vi "Teleop.vi"(10 "Match Info":T1={"Autonomous Elapsed Seconds"=0.0, "TeleOp Elapsed Seconds"=0.0, "Disabled Elapsed Seconds"=0.0, "Visited Autonomous"=FALSE, "Visited TeleOp"=FALSE, "Visited Disabled"=FALSE, "Autonomous Settings"={"Autonomous Style"=enum."Independent", "VI Refnum"=refnum}}, 11 "Call Context":T2) -> ()   [LabVIEW 2017]
doc: "This VI is called for each enabled TeleOp packet received from the DS. It is typically used to read from joysticks and other inputs and update I/O or setpoints for timed control loops. It should complete and return within 20 milliseconds or risk missing DS packets."
uses:
  <vilib>/Rock Robotics/WPI/DriverStation/WPI_DriverStationDerivedRobotMode.ctl
  <vilib>/Rock Robotics/WPI/DriverStation/WPI_DriverStationMatch Info.ctl
  <vilib>/Rock Robotics/WPI/Relay/WPI_RelayValue.ctl
  <vilib>/Rock Robotics/WPI/Solenoid/WPI_SolenoidValue.ctl
  <vilib>/Rock Robotics/WPI/Utilities/WPI_GetSetVariantRefNum.vi
  <vilib>/Rock Robotics/WPI/RobotDrive/WPI_RobotDriveMecanumDrive_Cartesian.vi
  <vilib>/Rock Robotics/WPI/Solenoid/WPI_SolenoidSetEnum.vi
panel:
  out "Distance":dbl
  out "Magnet sensed 2":bool
  out "Magnet sensed 1":bool
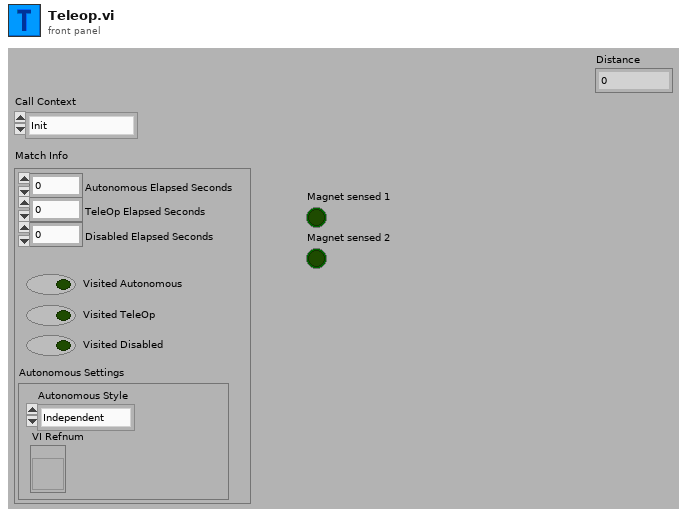
[diagram p1: front panel]
types:
  T1 = typedef "WPI_DriverStationMatch Info.ctl" = cluster{"Autonomous Elapsed Seconds":dbl, "TeleOp Elapsed Seconds":dbl, "Disabled Elapsed Seconds":dbl, "Visited Autonomous":bool, "Visited TeleOp":bool, "Visited Disabled":bool, "Autonomous Settings":cluster{"Autonomous Style":enum16{"Iterative", "Independent"}, "VI Refnum":refnum<vi>}}
  T2 = typedef "WPI_DriverStationDerivedRobotMode.ctl" = enum16{"Init", "Execute", "Stop"}
  T3 = typedef "WPI_SolenoidValue.ctl" = enum16{"Off", "On", "Forward", "Reverse"}
  T4 = typedef "WPI_RelayValue.ctl" = enum16{"Off", "On", "Forward", "Reverse"}
  T5 = typedef "WPI_CompressorDevRef.ctl" = cluster{"DevStatus":errorcluster, "Pneumatics Control Module":u8}
  T6 = typedef "WPI_EncoderDevRef.ctl" = cluster{"DevStatus":errorcluster, "EncoderIndex":T7, "CounterIndex":T8, "DistancePerCount":dbl, "Decoding Type":T9}
  T7 = typedef "FPGA_EncoderIdx.ctl" = enum8{"Enc 0", "Enc 1", "Enc 2", "Enc 3", "Enc 4", "Enc 5", "Enc 6", "Enc 7", "Invalid"}
  T8 = typedef "FPGA_CounterCtrSystemIndex.ctl" = enum8{"Ctr 0", "Ctr 1", "Ctr 2", "Ctr 3", "Ctr 4", "Ctr 5", "Ctr 6", "Ctr 7", "Invalid"}
  T9 = typedef "WPI_EncoderType.ctl" = enum16{"1x", "2x", "4x"}
  T10 = typedef "WPI_DigitalInputDevRef.ctl" = cluster{"DevStatus":errorcluster, "DIO Channel":T11}
  T11 = typedef "FPGA_DIOChannel.ctl" = enum8{"DIO 0", "DIO 1", "DIO 2", "DIO 3", "DIO 4", "DIO 5", "DIO 6", "DIO 7", "DIO 8", "DIO 9", "DIO MXP 0", "DIO MXP 1", "DIO MXP 2", "DIO MXP 3", "DIO MXP 4", "DIO MXP 5", "DIO MXP 6", "DIO MXP 7", "DIO MXP 8", "DIO MXP 9", "DIO MXP 10", "DIO MXP 11", "DIO MXP 12", "DIO MXP 13", "DIO MXP 14", "DIO MXP 15", "SPI Port CS1", "SPI Port CS2", "SPI Port CS3", "SPI Port MISO", "SPI Port MOSI", "Invalid"}
  T12 = typedef "WPI_RobotDriveDevRef.ctl" = cluster{"DevStatus":errorcluster, "Motors[]":T13[], "Square Inputs":bool, "Max Output":dbl}
  T13 = typedef "WPI_MotorControlDeviceRef.ctl" = cluster{"DeviceStatus":errorcluster, "Type":T14, "PWM":cluster{"PWM Channel":T15, "DeadBand":T16}, "CAN":cluster{"Device Number":u8, "SetOutput VI Ref":variant, "GetOutput VI Ref":variant, "Enable VI Ref":variant, "Disable VI Ref":variant, "Data":variant}, "Invert":bool, "DIO PWM":cluster{"PWM \"Enable\" Channel":T15, "DIOChannel":T11, "PWM Rate":dbl}}
  T14 = typedef "WPI_MotorControlType.ctl" = enum16{"PWM", "CAN", "DIO PWM"}
  T15 = typedef "FPGA_DIOPWMChannel.ctl" = enum8{"PWM 0", "PWM 1", "PWM 2", "PWM 3", "PWM 4", "PWM 5", "PWM 6", "PWM 7", "PWM 8", "PWM 9", "PWM MXP 0", "PWM MXP 1", "PWM MXP 2", "PWM MXP 3", "PWM MXP 4", "PWM MXP 5", "PWM MXP 6", "PWM MXP 7", "PWM MXP 8", "PWM MXP 9", "Invalid"}
  T16 = typedef "WPI_PWMDeadband.ctl" = cluster{"Name":string, "maxPositivePwm":i32, "minPositivePwm":i32, "centerPwm":i32, "maxNegativePwm":i32, "minNegativePwm":i32, "angularRange":u16}
  T17 = typedef "WPI_JoystickDevRef.ctl" = cluster{"Device":T18}
  T18 = typedef "WPI_JoystickDeviceEnum.ctl" = enum16{"USB 0", "USB 1", "USB 2", "USB 3", "USB 4", "USB 5"}
  T19 = cluster{"Axes[0]":dbl, "Axes[1]":dbl, "Axes[2]":dbl, "Axes[3]":dbl, "Axes[4]":dbl, "Axes[5]":dbl, "Axes[6]":dbl, "Axes[7]":dbl, "Axes[8]":dbl}
  T20 = cluster{"Buttons[0]":bool, "Buttons[1]":bool, "Buttons[2]":bool, "Buttons[3]":bool, "Buttons[4]":bool, "Buttons[5]":bool, "Buttons[6]":bool, "Buttons[7]":bool, "Buttons[8]":bool}
  T21 = typedef "WPI_RelayDevRef.ctl" = cluster{"DevStatus":errorcluster, "Relay Channel":T22, "Relay Direction":T23}
  T22 = typedef "FPGA_DIORelayChannel.ctl" = enum8{"Relay 0", "Relay 1", "Relay 2", "Relay 3", "Invalid"}
  T23 = typedef "WPI_RelayDirection.ctl" = enum16{"Both directions", "Forward only", "Reverse only"}
  T24 = typedef "WPI_SolenoidDevRef.ctl" = cluster{"DevStatus":errorcluster, "Pneumatics Control Module":u8, "Forward Solenoid Channel":T25, "Reverse Solenoid Channel":T25}
  T25 = typedef "WPI_SolenoidChannel.ctl" = enum8{"Solenoid 0", "Solenoid 1", "Solenoid 2", "Solenoid 3", "Solenoid 4", "Solenoid 5", "Solenoid 6", "Solenoid 7", "Invalid"}
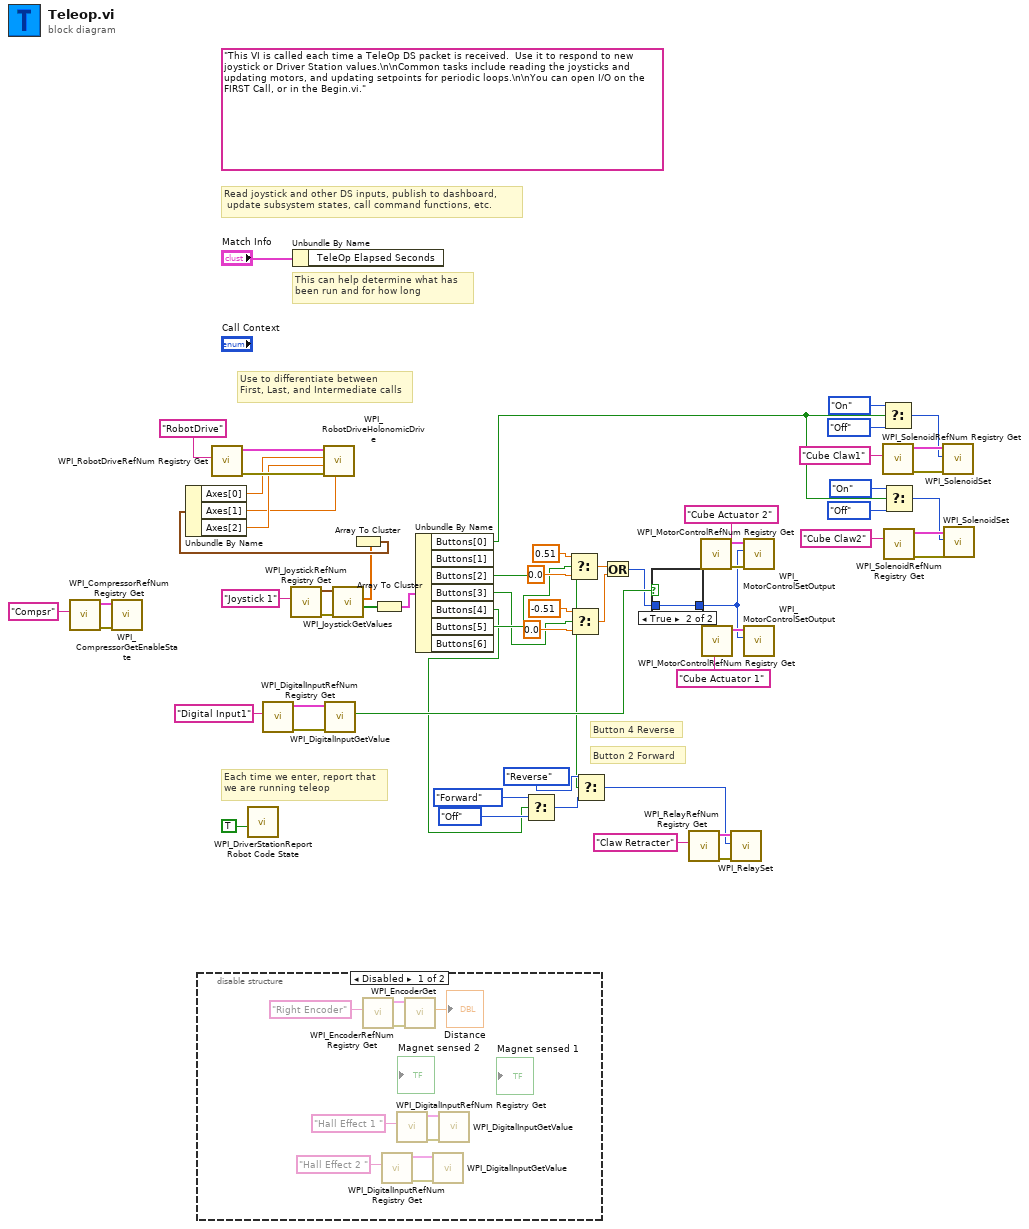
[diagram p0: block diagram]
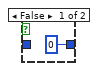
[diagram p2: hidden frame]
diagram:
  (unwired) "This VI is called each time a TeleOp DS packet is received.  Use it to respond to new joystick or Driver Station values.\n\nCommon tasks include reading the joysticks and updating motors, and updating setpoints for periodic loops.\n\nYou can open I/O on the FIRST Call, or in the Begin.vi."
  # "Button 2 Forward"
  # "Button 4 Reverse"
  # "Read joystick and other DS inputs, publish to dashboard,\n update subsystem states, call command functions, etc."
  # "Each time we enter, report that\nwe are running teleop"
  # "Use to differentiate between\nFirst, Last, and Intermediate calls"
  # "This can help determine what has\nbeen run and for how long"
  n1 = call <vilib>:"WPI_CompressorRefNum Registry Get.vi"("refnum name"="Compsr") -> ("error out"=w4:errorcluster, "CompressorDevRef"=w3:T5)  [unwired: 9 in]
  n2 = call <vilib>:"WPI_CompressorGetEnableState.vi"("error in (no error)"=w4, "CompressorDevRef"=w3) -> ()  [unwired: 6 in, 4 out]
  n3 = disable-structure shown="Disabled" {
    frame Disabled {
      n4 = call <vilib>:"WPI_EncoderRefNum Registry Get.vi"("refnum name"="Right Encoder") -> ("error out"=w69:errorcluster, "EncoderDevRef"=w70:T6)  [unwired: 9 in]
      n5 = call <vilib>:"WPI_DigitalInputRefNum Registry Get.vi"("refnum name"="Hall Effect 2 ") -> ("error out"=w66:errorcluster, "DigitalInputDevRef"=w65:T10)  [unwired: 9 in]
      n6 = call <vilib>:"WPI_DigitalInputRefNum Registry Get.vi"("refnum name"="Hall Effect 1 ") -> ("error out"=w64:errorcluster, "DigitalInputDevRef"=w63:T10)  [unwired: 9 in]
      n7 = call <vilib>:"WPI_EncoderGet.vi"("error in (no error)"=w69, "EncoderDevRef"=w70) -> ("Distance"=→"Distance":dbl)  [unwired: 4 in, 5 out]
      n8 = call <vilib>:"WPI_DigitalInputGetValue.vi"("error in (no error)"=w66, "DigitalInputDevRef"=w65) -> ()  [unwired: 7 in, 3 out]
      n9 = call <vilib>:"WPI_DigitalInputGetValue.vi"("error in (no error)"=w64, "DigitalInputDevRef"=w63) -> ()  [unwired: 7 in, 3 out]
    }
    frame Enabled {
    }
  }
  n10 = call <vilib>:"WPI_RobotDriveRefNum Registry Get.vi"("refnum name"="RobotDrive") -> ("error out"=w56:errorcluster, "RobotDriveDevRef"=w57:T12)  [unwired: 9 in]
  n11 = call <vilib>:"WPI_DriverStationReport Robot Code State.vi"("TeleOp"=TRUE ("Autonomous")) -> ()  [unwired: 10 in, 1 out]
  n12 = call <vilib>:"WPI_DigitalInputRefNum Registry Get.vi"("refnum name"="Digital Input1") -> ("error out"=w34:errorcluster, "DigitalInputDevRef"=w36:T10)  [unwired: 9 in]
  n13 = call <vilib>:"WPI_JoystickRefNum Registry Get.vi"("refnum name"="Joystick 1") -> ("error out"=w55:errorcluster, "JoystickDevRef"=w54:T17)  [unwired: 9 in]
  n14 = Unbundle By Name("Match Info") -> ()  [unwired: 1 out]
  n15 = call <vilib>:"WPI_DigitalInputGetValue.vi"("error in (no error)"=w34, "DigitalInputDevRef"=w36) -> ("Value"=w32:bool)  [unwired: 7 in, 2 out]
  n16 = call <vilib>:"WPI_JoystickGetValues.vi"("error in (no error)"=w55, "JoystickDevRef"=w54) -> ("Buttons"=w52:bool[], "Axes"=w42:dbl[])  [unwired: 5 in, 3 out]
  n17 = Array To Cluster(array=w42) -> (cluster=w43:T19)
  n18 = Unbundle By Name(w43) -> ("Axes[0]"=w41:dbl, "Axes[1]"=w39:dbl, "Axes[2]"=w40:dbl)
  n19 = call-poly <vilib>:"WPI_RobotDriveHolonomicDrive.vi"("Rotation"=w39, "error in (no error)"=w56, "Y"=w40, "X"=w41, "RobotDriveDevRef"=w57) -> ()  [unwired: 4 in, 3 out]
  n20 = Array To Cluster(array=w52) -> (cluster=w51:T20)
  n21 = Unbundle By Name(w51) -> ("Buttons[0]"=w7:bool, "Buttons[2]"=w20:bool, "Buttons[3]"=w29:bool, "Buttons[4]"=w21:bool, "Buttons[5]"=w30:bool)  [unwired: 2 out]
  n22 = Select(t=WPI_RelayValue."Forward" ("RelayValue"), s=w21, f=WPI_RelayValue."Off" ("RelayValue")) -> (s? t:f=w28:T4)
  n23 = Select(t=0.51, s=w30, f=0.0) -> (s? t:f=w33:dbl)
  n24 = Select(t=-0.51, s=w29, f=0.0) -> (s? t:f=w44:dbl)
  n25 = Select(t=WPI_RelayValue."Reverse" ("RelayValue"), s=w20, f=w28) -> (s? t:f=w1:T4)
  n26 = Or(x=w33, y=w44) -> (x .or. y?=w31:i32)
  n27 = case shown="True" w32 {
    tunnel: w31 -> [_ w72]
    tunnel: [0 w72] -> w5
    frame False {
    }
    frame True {
    }
  }
  n28 = call <vilib>:"WPI_RelayRefNum Registry Get.vi"("refnum name"="Claw Retracter") -> ("error out"=w24:errorcluster, "RelayDevRef"=w23:T21)  [unwired: 9 in]
  n29 = call <vilib>:"WPI_MotorControlRefNum Registry Get.vi"("refnum name"="Cube Actuator 2") -> ("error out"=w50:errorcluster, "MotorControlDevRef"=w49:T13)  [unwired: 9 in]
  n30 = call <vilib>:"WPI_MotorControlRefNum Registry Get.vi"("refnum name"="Cube Actuator 1") -> ("MotorControlDevRef"=w38:T13)  [unwired: 9 in, 1 out]
  n31 = call <vilib>:"WPI_RelaySet.vi"("error in (no error)"=w24, "RelayValue"=w1, "RelayDevRef"=w23) -> ()  [unwired: 7 in, 2 out]
  n32 = call <vilib>:"WPI_MotorControlSetOutput.vi"("error in (no error)"=w50, "Output"=w5, "MotorControlDevRef"=w49) -> ()  [unwired: 6 in, 3 out]
  n33 = call <vilib>:"WPI_MotorControlSetOutput.vi"("Output"=w5, "MotorControlDevRef"=w38) -> ()  [unwired: 7 in, 3 out]
  n34 = Select(t=WPI_SolenoidValue."On" ("Value"), s=w7, f=WPI_SolenoidValue."Off" ("Value")) -> (s? t:f=w17:T3)
  n35 = call <vilib>:"WPI_SolenoidRefNum Registry Get.vi"("refnum name"="Cube Claw1") -> ("error out"=w18:errorcluster, "SolenoidDevRef"=w19:T24)  [unwired: 9 in]
  n36 = Select(t=WPI_SolenoidValue."On" ("Value"), s=w7, f=WPI_SolenoidValue."Off" ("Value")) -> (s? t:f=w11:T3)
  n37 = call <vilib>:"WPI_SolenoidRefNum Registry Get.vi"("refnum name"="Cube Claw2") -> ("error out"=w13:errorcluster, "SolenoidDevRef"=w12:T24)  [unwired: 9 in]
  n38 = call-poly <vilib>:"WPI_SolenoidSet.vi"("error in (no error)"=w18, "Value"=w17, "SolenoidDevRef"=w19) -> ()  [unwired: 7 in, 2 out]
  n39 = call-poly <vilib>:"WPI_SolenoidSet.vi"("error in (no error)"=w13, "Value"=w11, "SolenoidDevRef"=w12) -> ()  [unwired: 7 in, 2 out]
